vi "Sensor Loop.vi"() -> ()   [LabVIEW 2014, in "Elevator System.lvlib"]
uses:
  Elevator System.lvlib
  SimulatorVIs/Simulation Input Global.vi
  Typedef/FGVAction.ctl
  <vilib>/ptbypt/NI_PtbyPt.lvlib
panel:
  in  "elevators parameters":T1={"static gain"=10.0, "lag (s)"=0.05, "deadtime (s)"=0.01, "load"=0.0, "deadband"=0.0, "sensor noise"=0.0, "initial PV"=6.0, "plant noise"=0.0} {"plant noise" format="%.2f"; "initial PV" format="%.2f"; "sensor noise" format="%.2f"; "lag (s)" format="%.2f"; "deadtime (s)" format="%.2f"; "deadband" format="%.1f"; "load" format="%.2f"; "static gain" format="%.2f"}
  in  "gripper parameters":T1={"static gain"=2.5, "lag (s)"=2.5, "deadtime (s)"=0.01, "load"=40.0, "deadband"=0.0, "sensor noise"=0.0, "initial PV"=0.0, "plant noise"=0.0} {"plant noise" format="%.2f"; "initial PV" format="%.2f"; "sensor noise" format="%.2f"; "lag (s)" format="%.2f"; "deadtime (s)" format="%.2f"; "deadband" format="%.1f"; "load" format="%.2f"; "static gain" format="%.2f"}
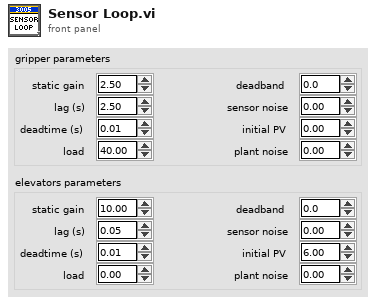
[diagram p1: front panel]
types:
  T1 = cluster{"static gain":dbl, "lag (s)":dbl, "deadtime (s)":dbl, "load":dbl, "deadband":dbl, "sensor noise":dbl, "initial PV":dbl, "plant noise":dbl}
  T2 = typedef "Elevator System.lvlib/FGVAction.ctl" = enum16{"get", "set"}
  T3 = typedef "WPI_PotentiometerDevRef.ctl" = cluster{"DevStatus":errorcluster, "Controller":T4, "Analog Channel":T5, "Invert Output":bool}
  T4 = typedef "FPGA_TypedefAnalogModule.ctl" = enum16{"Controller 1"}
  T5 = typedef "FPGA_AIChannel.ctl" = enum8{"AI 0", "AI 1", "AI 2", "AI 3", "AI MXP 0", "AI MXP 1", "AI MXP 2", "AI MXP 3", "Invalid"}
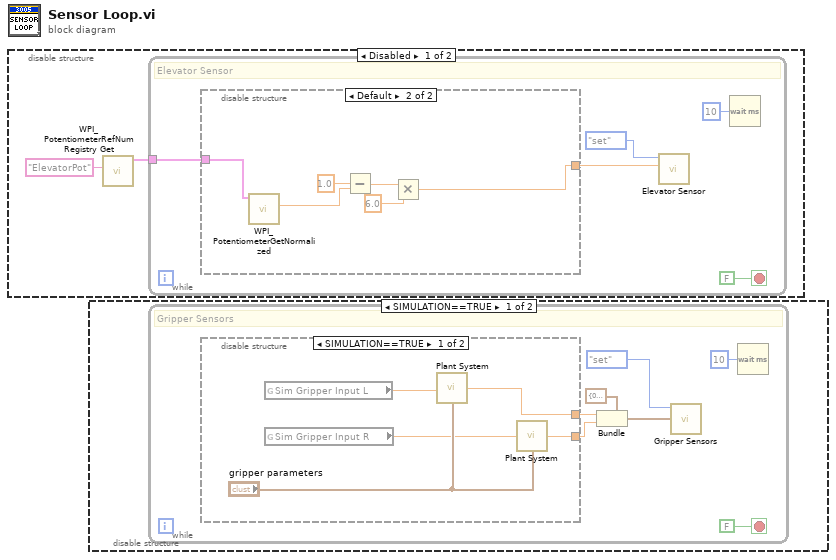
[diagram p0: block diagram]
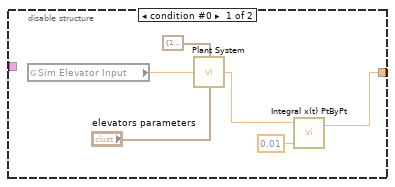
[diagram p2: hidden frame]
diagram:
  n1 = disable-structure shown="Disabled" {
    frame Disabled {
      n2 = call <vilib>:"WPI_PotentiometerRefNum Registry Get.vi"("refnum name"="ElevatorPot") -> ("PotDevRef"=w1:T3)  [unwired: 9 in, 1 out]
      n3 = while {
        tunnel: w1 -> [w3]
        stop <- FALSE stop-if-true
        # "Elevator Sensor"
        n4 = disable-structure shown="Default" {
          disable-tunnel: [w9 w14] -> w4
          disable-tunnel: w3 -> [_ w15]
          frame condition #0 {
            n5 = global read "Simulation Input Global.vi" "Sim Elevator Input"() -> (w12:dbl)
            n6 = call "Plant System.vi"("output saturation range"=cluster{"output high":dbl, "output low":dbl} {"output high"=100.0, "output low"=-100.0}, "Plant Input"=w12, "process parameters"="elevators parameters") -> ("Plant Output"=w10:dbl)  [unwired: 12 in]
            n7 = call <vilib>:"Integral x(t) PtByPt.vi"("dt"=0.01, "x"=w10) -> ("integral x(t)"=w9:dbl)  [unwired: 2 in, 1 out]
          }
          frame condition #1 (active) {
            n8 = call <vilib>:"WPI_PotentiometerGetNormalized.vi"("PotDevRef"=w15) -> ("Normalized Value"=w16:dbl)  [unwired: 8 in, 2 out]
            n9 = Subtract(x=1.0, y=w16) -> (x-y=w18:dbl)
            n10 = Multiply(x=w18, y=6.0) -> (x*y=w14:dbl)
          }
        }
        n11 = call "Elevator Sensor.vi"("Value"=w4, "Action"=FGVAction."set") -> ()  [unwired: 8 in, 2 out]
        n12 = Wait (ms)(milliseconds to wait=u32 10) -> ()  [unwired: 1 out]
      }
    }
    frame Enabled {
    }
  }
  n13 = disable-structure shown="SIMULATION==TRUE" {
    frame condition #0 {
      n14 = while {
        stop <- FALSE stop-if-true
        # "Gripper Sensors"
        n15 = disable-structure shown="SIMULATION==TRUE" {
          disable-tunnel: [w28 _] -> w23
          disable-tunnel: [w27 _] -> w22
          frame condition #0 {
            n16 = global read "Simulation Input Global.vi" "Sim Gripper Input L"() -> (w30:dbl)
            n17 = global read "Simulation Input Global.vi" "Sim Gripper Input R"() -> (w29:dbl)
            n18 = call "Plant System.vi"("Plant Input"=w30, "process parameters"="gripper parameters") -> ("Plant Output"=w28:dbl)  [unwired: 13 in]
            n19 = call "Plant System.vi"("Plant Input"=w29, "process parameters"="gripper parameters") -> ("Plant Output"=w27:dbl)  [unwired: 13 in]
          }
          frame condition #1 (active) {
          }
        }
        n20 = Bundle(cluster=cluster{"Left":dbl, "Right":dbl} {"Left"=0.0, "Right"=0.0} ("Gripper Values"), "Left"=w23, "Right"=w22) -> (w20:cluster{"Left":dbl, "Right":dbl})
        n21 = call "Gripper Sensors.vi"("Input"=w20, "Action"=FGVAction."set") -> ()  [unwired: 8 in, 2 out]
        n22 = Wait (ms)(milliseconds to wait=u32 10) -> ()  [unwired: 1 out]
      }
    }
    frame condition #1 (active) {
    }
  }
